vi "Configure Single Piece Mass.vi"(8 "error in (no error)":errorcluster, 10 "Single Piece Weight [g]":dbl=1.0, 11 "VISA resource name":refnum<visa-resource-name>) -> (0 "error out":errorcluster, 3 "VISA resource name out":refnum<visa-resource-name>)   [LabVIEW 2017, in "RadWag balances and scales.lvlib"]
doc: "Sets the value of single piece weight in counting mode.\nThis VI works properly when balance works in counting mode. (To configure work mode use Utility -> Set work mode)\nTo see proper usage of piece couting mode open Examples ->RadWag Counting Pieces"
uses:
  <instrlib>/Prev/RadWag Continuous Read Folder/RadWag balances and scales.lvlib
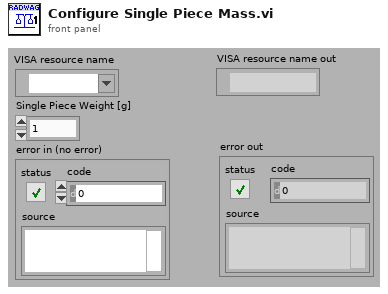
[diagram p1: front panel]
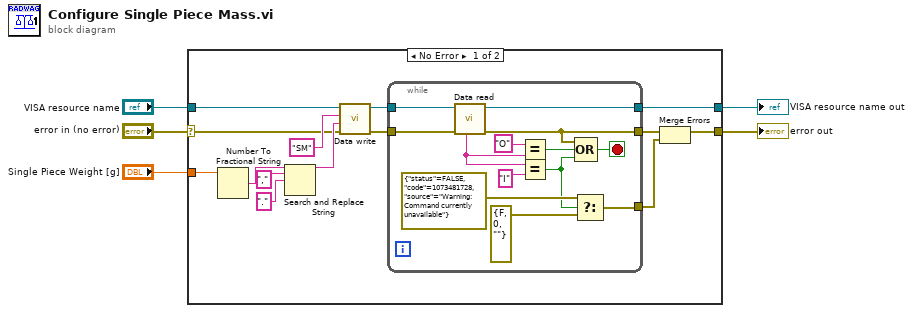
[diagram p0: block diagram]
diagram:
  n1 = case shown="No Error" "error in (no error)" {
    selector: "error in (no error)" -> [w10 w33]
    tunnel: "VISA resource name" -> [w19 w34]
    tunnel: [w17 w34] -> w4
    tunnel: [w6 w33] -> w3
    tunnel: "Single Piece Weight [g]" -> [w15 _]
    frame No Error {
      n2 = Number To Fractional String(number=w15) -> (F-format string=w14:string)  [unwired: 3 in]
      n3 = Search and Replace String(input string=w14, search string=",", replace string="." ("replace string (\"\")")) -> (result string=w11:string)  [unwired: 5 in, 3 out]
      n4 = call <instrlib>:"Data write.vi"("error in (no error)"=w10, "Parameter"=w11, "ID"="SM", "VISA resource name"=w19) -> ("error out"=w9:errorcluster, "VISA resource name out"=w18:refnum<visa-resource-name>)  [unwired: 6 in]
      n5 = while {
        tunnel: w18 -> [w32]
        tunnel: [w31] -> w17
        tunnel: [w25] -> w8
        tunnel: w9 -> [w26]
        tunnel: [w20] -> w7
        stop <- w27 stop-if-true
        n6 = call <instrlib>:"Data read.vi"("error in (no error)"=w26, "VISA resource name"=w32) -> ("error out"=w25:errorcluster, "VISA resource name out"=w31:refnum<visa-resource-name>, "Status"=w30:string)  [unwired: 3 in, 4 out]
        n7 = Equal?(x="O", y=w30) -> (x = y?=w24:bool)
        n8 = Equal?(x=w30, y="I") -> (x = y?=w21:bool)
        n9 = Compound Arithmetic op=OR(w25, w24, w21) -> (w27:bool)
        n10 = Select(t=errorcluster {"status"=FALSE, "code"=1073481728, "source"="Warning: Command currently unavailable"}, s=w21, f=errorcluster {"status"=FALSE, "code"=0, "source"=""} ("error constant")) -> (s? t:f=w20:errorcluster)
      }
      n11 = Merge Errors(w8, w7) -> (w6:errorcluster)
    }
    frame Error {
    }
  }
  "VISA resource name out" <- w4
  "error out" <- w3
